vi "Playback Controls.vi"() -> ()   [LabVIEW 2014]
uses:
  <vilib>/Rock Robotics/WPI/Dashboard/WPI_DashboardPlay Operation.ctl
  <vilib>/Rock Robotics/WPI/Dashboard/WPI_DashboardLogging Global.vi
  <vilib>/Utility/inputDevices.llb/mouseAcquire.vi
panel:
  in  "Operation":u16(ring) items=["", "Rename", "Delete", "Show Folder"]
  in  "Rename":string
  in  "Dragging?":bool
  in  "Scrollbar":dbl(slide) scale=0.0..3.043
  in  "Speed":u16(ring)=3 items=["1/10 x", "1/5 x", "1/2 x", "1 x", "2 x", "5 x", "10 x"]
  in  "Playback Button":bool
  in  "Pause Button":bool
  in  "File Selector":u16(ring) items=["Select a Log File", "2013_08_04 10_32_21 Sun -- 1.2 secs", "2013_08_04 10_32_23 Sun -- 0.6 secs", "2013_08_04 10_32_25 Sun -- 0.6 secs", "2013_08_04 10_32_26 Sun -- 0.5 secs", "2013_08_04 10_32_28 Sun -- 0.7 secs", "2013_08_04 10_32_29 Sun -- 0.7 secs", "2013_08_04 10_32_31 Sun -- 0.5 secs", "2013_08_04 10_32_32 Sun -- 14.4 secs", "bar -- 2.2 secs", "foo -- 3.0 secs"]
  in  "Drag Button":bool
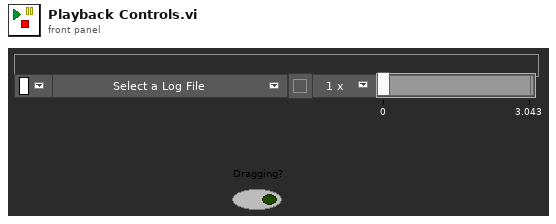
[diagram p1: front panel]
types:
  T1 = typedef "WPI_DashboardPlay Operation.ctl" = enum16{"Play", "Pause", "Finished"}
  T2 = typedef "LVRectTypeDef.ctl" = cluster{"Left":i16, "Top":i16, "Right":i16, "Bottom":i16}
  T3 = cluster{"Horizontal":i32, "Vertical":i32, "Scrolling":i32}
  T4 = cluster{"Horizontal":i32, "Vertical":i32, "Horizontal":i32, "Vertical":i32}
  T5 = cluster{"button 1":bool, "button 2":bool, "button 3":bool, "button 4":bool}
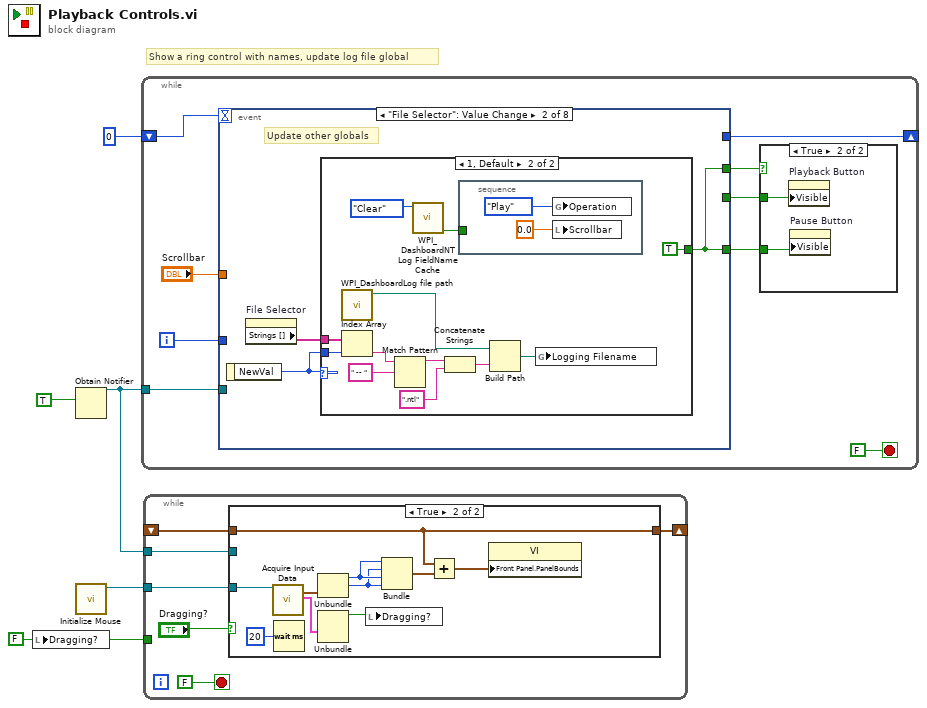
[diagram p0: block diagram]
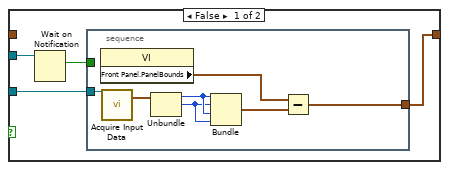
[diagram p2: hidden frame]
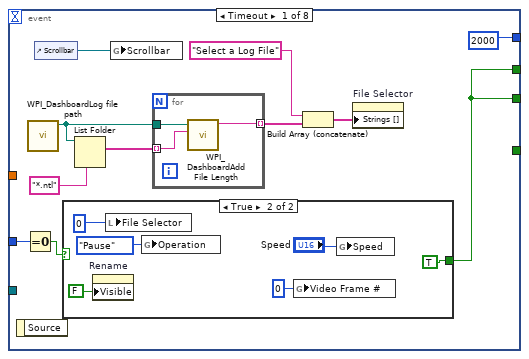
[diagram p4: hidden frame]
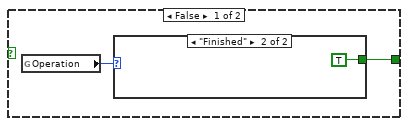
[diagram p5: hidden frame]
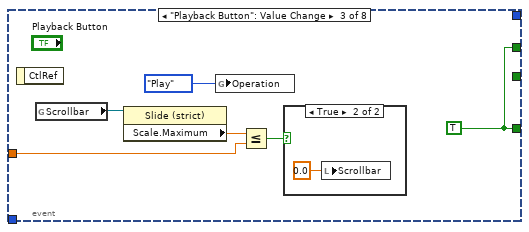
[diagram p8: hidden frame]
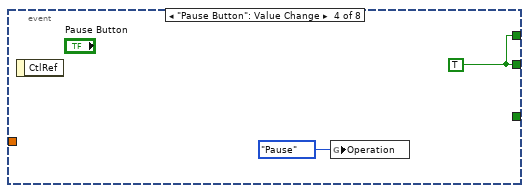
[diagram p10: hidden frame]
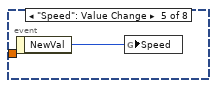
[diagram p11: hidden frame]
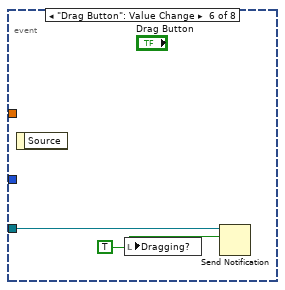
[diagram p12: hidden frame]
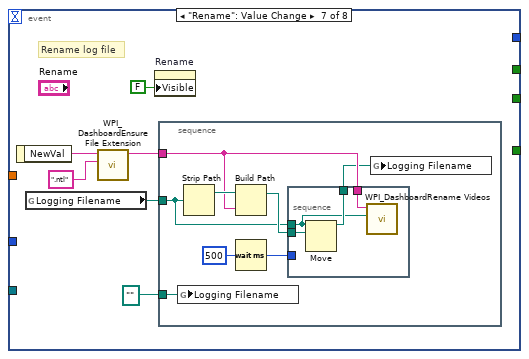
[diagram p13: hidden frame]
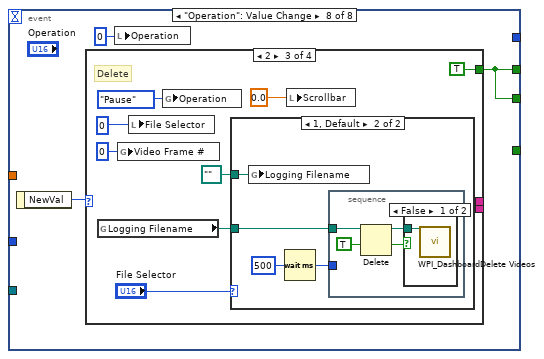
[diagram p14: hidden frame]
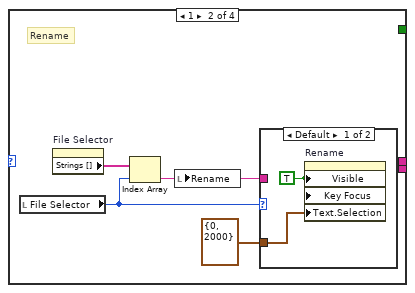
[diagram p16: hidden frame]
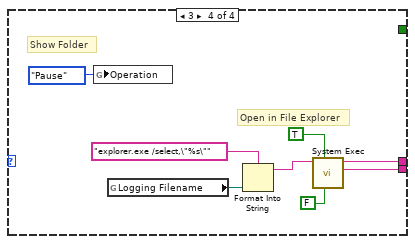
[diagram p20: hidden frame]
diagram:
  w2 = FALSE ("Dragging?")
  # "Show a ring control with names, update log file global"
  n1 = local write "Dragging?"(w2) -> ()
  n2 = Obtain Notifier(notification data type=TRUE ("Dragging?")) -> (notifier out=w3:refnum<notifier>)  [unwired: 3 in, 2 out]
  n3 = call <vilib>:"Initialize Mouse.vi"() -> ("device ID"=w4:refnum<k1>)  [unwired: 10 in, 1 out]
  n4 = while {
    shift-right: [w13] -> _
    shift-left: 0 -> [w12]
    tunnel: w3 -> [w6]
    i -> [w8]
    stop <- FALSE stop-if-true
    n5 = event shown="[1] \"File Selector\": Value Change" {
      selector: _ -> [_ _ _ _ _ _ _ _]
      dyn-events: _ -> [_ _ _ _ _ _ _ _]
      timeout: w12 -> [_ _ _ _ _ _ _ _]
      tunnel: [2000 _ _ _ _ _ _ _] -> w13
      tunnel: [_ w40 w62 _ _ _ _ _] -> w11
      tunnel: [w18 _ _ w65 _ _ _ w88] -> w10
      tunnel: [w18 w40 w62 w65 _ _ _ w88] -> w9
      tunnel: w8 -> [w20 _ _ _ _ _ _ _]
      tunnel: "Scrollbar" -> [_ _ w58 _ _ _ _ _]
      tunnel: w6 -> [_ _ _ _ _ w68 _ _]
      event Timeout {
        n6 = event-data() -> ()  [unwired: 1 in, 1 out]
        n7 = Equal To 0?(x=w20) -> (x = 0?=w19:bool)
        n8 = call <vilib>:"WPI_DashboardLog file path.vi"() -> ("appended path"=w17:path)  [unwired: 11 in]
        n9 = control-ref of="Scrollbar"() -> (w24:refnum<vi>)
        n10 = case shown="True" w19 {
          tunnel: [w28 TRUE] -> w18
          frame False {
            n11 = global read "WPI_DashboardLogging Global.vi" "Operation"() -> (w29:T1)
            n12 = case shown="\"Finished\"" w29 {
              tunnel: [_ TRUE] -> w28
              frame Default {
              }
              frame "Finished" {
              }
            }
          }
          frame True {
            n13 = property on="Rename" class="Str"("Visible"=FALSE) -> ()  [unwired: 2 in, 2 out]
            n14 = local write "File Selector"(0) -> ()
            n15 = global write "WPI_DashboardLogging Global.vi" "Operation"(WPI_DashboardPlay_Operation."Pause" ("Operation")) -> ()
            n16 = global write "WPI_DashboardLogging Global.vi" "Video Frame #"(0 ("Video Frame #")) -> ()
            n17 = global write "WPI_DashboardLogging Global.vi" "Speed"("Speed") -> ()
          }
        }
        n18 = List Folder(path=w17, pattern="*.ntl") -> (filenames=w26:string[])  [unwired: 2 in, 3 out]
        n19 = global write "WPI_DashboardLogging Global.vi" "Scrollbar"(w24) -> ()
        n20 = for {
          tunnel: w26 -> [w37] mode=indexing
          tunnel: [w39] -> w23 mode=indexing
          tunnel: w17 -> [w38]
          n21 = call <vilib>:"WPI_DashboardAdd File Length.vi"("String in"=w37, "appended path"=w38) -> ("String out"=w39:string)  [unwired: 9 in]
        }
        n22 = Build Array (concatenate)("Select a Log File" ("pattern"), w23) -> (w22:string[])
        n23 = property on="File Selector" class="Ring (strict)"("Strings []"=w22) -> ()  [unwired: 2 in, 2 out]
      }
      event "File Selector": Value Change {
        # "Update other globals"
        n24 = event-data() -> ("NewVal"=w41:u16)  [unwired: 1 in]
        n25 = property on="File Selector" class="Ring (strict)"() -> ("Strings []"=w42:string[])  [unwired: 2 in, 2 out]
        n26 = case shown="1, Default" w41 {
          tunnel: w42 -> [_ w54]
          tunnel: w41 -> [_ w53]
          tunnel: [_ TRUE ("Visible")] -> w40
          frame 0 {
          }
          frame 1, Default {
            n27 = call <vilib>:"WPI_DashboardLog file path.vi"() -> ("appended path"=w52:path)  [unwired: 11 in]
            n28 = Index Array(array=w54, index=w53) -> (element=w48:string)
            n29 = Match Pattern(string=w48, regular expression=" -- ") -> (before substring=w43:string)  [unwired: 1 in, 3 out]
            n30 = call <vilib>:"WPI_DashboardNT Log FieldName Cache.vi"("Operation"=enum16{"Lookup/Add", "Index", "Clear"}."Clear") -> ("New/Valid"=w45:bool)  [unwired: 8 in, 2 out]
            n31 = Concatenate Strings(w43, ".ntl") -> (w50:string)
            n32 = stacked-sequence {
              tunnel: w45 -> [_]
              frame #0 {
                n33 = global write "WPI_DashboardLogging Global.vi" "Operation"(WPI_DashboardPlay_Operation."Play" ("Operation")) -> ()
                n34 = local write "Scrollbar"(0.0 ("Position")) -> ()
              }
            }
            n35 = Build Path(base path=w52, name or relative path=w50) -> (appended path=w49:path)
            n36 = global write "WPI_DashboardLogging Global.vi" "Logging Filename"(w49) -> ()
          }
        }
      }
      event "Playback Button": Value Change {
        w62 = TRUE ("Visible")
        n37 = event-data() -> ()  [unwired: 1 in, 1 out]
        n38 = global read "WPI_DashboardLogging Global.vi" "Scrollbar"() -> (w60:refnum<vi>)
        n39 = property class="Slide (strict)"(reference=w60) -> ("Scale.Maximum"=w59:dbl)  [unwired: 1 in, 2 out]
        n40 = global write "WPI_DashboardLogging Global.vi" "Operation"(WPI_DashboardPlay_Operation."Play" ("Operation")) -> ()
        n41 = Less Or Equal?(x=w59, y=w58) -> (x <= y?=w57:bool)
        n42 = case shown="True" w57 {
          frame False {
          }
          frame True {
            n43 = local write "Scrollbar"(0.0 ("Scrollbar")) -> ()
          }
        }
      }
      event "Pause Button": Value Change {
        w65 = TRUE ("Visible")
        n44 = event-data() -> ()  [unwired: 1 in, 1 out]
        n45 = global write "WPI_DashboardLogging Global.vi" "Operation"(WPI_DashboardPlay_Operation."Pause" ("Operation")) -> ()
      }
      event "Speed": Value Change {
        n46 = event-data() -> ("NewVal"=w66:u16)  [unwired: 1 in]
        n47 = global write "WPI_DashboardLogging Global.vi" "Speed"(w66) -> ()
      }
      event "Drag Button": Value Change {
        w67 = TRUE ("Dragging?")
        n48 = event-data() -> ()  [unwired: 1 in, 1 out]
        n49 = local write "Dragging?"(w67) -> ()
        n50 = Send Notification(notification=w67, notifier=w68) -> ()  [unwired: 1 in, 2 out]
      }
      event "Rename": Value Change {
        # "Rename log file"
        n51 = event-data() -> ("NewVal"=w71:string)  [unwired: 1 in]
        n52 = global read "WPI_DashboardLogging Global.vi" "Logging Filename"() -> (w73:path)
        n53 = call <vilib>:"WPI_DashboardEnsure File Extension.vi"("Extension"=".ntl", "Name"=w71) -> ("Name Out"=w70:string)  [unwired: 9 in]
        n54 = property on="Rename" class="Str"("Visible"=FALSE) -> ()  [unwired: 2 in, 2 out]
        n55 = stacked-sequence {
          tunnel: w70 -> [w76]
          tunnel: w73 -> [w80]
          tunnel: path "" ("Logging Filename") -> [w79]
          frame #0 {
            n56 = global write "WPI_DashboardLogging Global.vi" "Logging Filename"(w79) -> ()
            n57 = Strip Path(path=w80) -> (stripped path=w82:path)  [unwired: 1 out]
            n58 = Build Path(base path=w82, name or relative path=w76) -> (appended path=w81:path)
            n59 = Wait (ms)(milliseconds to wait=u32 500) -> (millisecond timer value=w77:u32)
            n60 = stacked-sequence {
              tunnel: w81 -> [w86]
              tunnel: w80 -> [w83]
              tunnel: w77 -> [_]
              tunnel: w76 -> [w85]
              tunnel: [w84] -> w75
              frame #0 {
                n61 = Move(source path=w83, 10:w86) -> (3:w84:path)  [unwired: 3 in, 2 out]
                n62 = call <vilib>:"WPI_DashboardRename Videos.vi"("Path"=w83, "Log Name"=w85) -> ()  [unwired: 10 in]
              }
            }
            n63 = global write "WPI_DashboardLogging Global.vi" "Logging Filename"(w75) -> ()
          }
        }
      }
      event "Operation": Value Change {
        n64 = event-data() -> ("NewVal"=w89:u16)  [unwired: 1 in]
        n65 = case shown="2" w89 {
          tunnel: [_ _ TRUE _] -> w88
          tunnel: [_ _ _ w116] -> _
          tunnel: [_ _ _ w115] -> _
          frame 0, Default {
          }
          frame 1 {
            # "Rename"
            n66 = local read "File Selector"() -> (w91:u16)
            n67 = property on="File Selector" class="Ring (strict)"() -> ("Strings []"=w93:string[])  [unwired: 2 in, 2 out]
            n68 = Index Array(array=w93, index=w91) -> (element=w92:string)
            n69 = local write "Rename"(w92) -> ()
            n70 = case shown="Default" w91 {
              tunnel: w92 -> [_ _]
              tunnel: cluster{i32, i32} {0, 2000} -> [w94 _]
              frame Default {
                w95 = TRUE ("Visible")
                n71 = property on="Rename" class="Str"("Visible"=w95, "Key Focus"=w95, "Text.Selection"=w94) -> ()  [unwired: 2 in, 2 out]
              }
              frame 0 {
              }
            }
          }
          frame 2 {
            # "Delete"
            n72 = global read "WPI_DashboardLogging Global.vi" "Logging Filename"() -> (w98:path)
            n73 = global write "WPI_DashboardLogging Global.vi" "Video Frame #"(0 ("Video Frame #")) -> ()
            n74 = local write "File Selector"(0) -> ()
            n75 = global write "WPI_DashboardLogging Global.vi" "Operation"(WPI_DashboardPlay_Operation."Pause" ("Operation")) -> ()
            n76 = case shown="1, Default" "File Selector" {
              tunnel: w98 -> [_ w107]
              tunnel: path "" ("Logging Filename") -> [_ w106]
              frame 0 {
              }
              frame 1, Default {
                n77 = global write "WPI_DashboardLogging Global.vi" "Logging Filename"(w106) -> ()
                n78 = Wait (ms)(milliseconds to wait=u32 500) -> (millisecond timer value=w104:u32)
                n79 = stacked-sequence {
                  tunnel: w107 -> [w111]
                  tunnel: w104 -> [_]
                  frame #0 {
                    n80 = Delete(path (use dialog)=w111, confirm (F)=TRUE) -> (deleted path=w108:path, cancelled=w109:bool)  [unwired: 3 in, 1 out]
                    n81 = case shown="False" w109 {
                      tunnel: w108 -> [w112 _]
                      frame False {
                        n82 = call <vilib>:"WPI_DashboardDelete Videos.vi"("Path"=w112) -> ()  [unwired: 11 in]
                      }
                      frame True {
                      }
                    }
                  }
                }
              }
            }
            n83 = local write "Scrollbar"(0.0 ("Position")) -> ()
          }
          frame 3 {
            # "Open in File Explorer"
            # "Show Folder"
            n84 = global write "WPI_DashboardLogging Global.vi" "Operation"(WPI_DashboardPlay_Operation."Pause" ("Operation")) -> ()
            n85 = global read "WPI_DashboardLogging Global.vi" "Logging Filename"() -> (w113:path)
            n86 = Format Into String(format string="explorer.exe /select,\"%s\"", w113) -> (resulting string=w119:string)  [unwired: 2 in, 1 out]
            n87 = call <vilib>:"System Exec.vi"("run minimized? (F)"=FALSE, "wait until completion? (T)"=TRUE, "command line"=w119) -> ("standard error"=w116:string, "standard output"=w115:string)  [unwired: 5 in, 2 out]
          }
        }
        n88 = local write "Operation"(0) -> ()
      }
    }
    n89 = case shown="True" w9 {
      tunnel: w11 -> [_ w16]
      tunnel: w10 -> [_ w15]
      frame False {
      }
      frame True {
        n90 = property on="Playback Button" class="Bool"("Visible"=w15) -> ()  [unwired: 2 in, 2 out]
        n91 = property on="Pause Button" class="Bool"("Visible"=w16) -> ()  [unwired: 2 in, 2 out]
      }
    }
  }
  n92 = while {
    tunnel: w4 -> [w126]
    tunnel: w3 -> [w124]
    tunnel: w2 -> [_]
    shift-right: [w122] -> _
    shift-left: _ -> [w121]
    stop <- FALSE stop-if-true
    n93 = case shown="True" "Dragging?" {
      tunnel: w126 -> [w129 w147]
      tunnel: w124 -> [w130 _]
      tunnel: [w128 w139] -> w122
      tunnel: w121 -> [_ w139]
      frame False {
        n94 = Wait on Notification(notifier=w130) -> (notification=w127:bool)  [unwired: 3 in, 3 out]
        n95 = stacked-sequence {
          tunnel: w129 -> [w137]
          tunnel: [w133] -> w128
          tunnel: w127 -> [_]
          frame #0 {
            n96 = property class="VI"() -> ("Front Panel.PanelBounds"=w135:T2)  [unwired: 2 in, 2 out]
            n97 = call-poly <vilib>:"Acquire Input Data.vi"("device ID"=w137) -> ("axis info"=w136:T3)  [unwired: 15 in, 3 out]
            n98 = Unbundle(w136) -> ("Horizontal"=w132:i32, "Vertical"=w131:i32)  [unwired: 1 out]
            n99 = Bundle("Horizontal"=w132, "Vertical"=w131, "Horizontal"=w132, "Vertical"=w131) -> (w134:T4)  [unwired: 1 in]
            n100 = Subtract(x=w135, y=w134) -> (x-y=w133:cluster{i32, i32, i32, i32})
          }
        }
      }
      frame True {
        n101 = call-poly <vilib>:"Acquire Input Data.vi"("device ID"=w147) -> ("axis info"=w143:T3, "button info"=w145:T5)  [unwired: 15 in, 2 out]
        n102 = Wait (ms)(milliseconds to wait=u32 20) -> ()  [unwired: 1 out]
        n103 = Unbundle(w143) -> ("Horizontal"=w142:i32, "Vertical"=w141:i32)  [unwired: 1 out]
        n104 = Unbundle(w145) -> ("button 1"=w144:bool)  [unwired: 3 out]
        n105 = local write "Dragging?"(w144) -> ()
        n106 = Bundle("Horizontal"=w142, "Vertical"=w141, "Horizontal"=w142, "Vertical"=w141) -> (w140:T4)  [unwired: 1 in]
        n107 = Add(x=w139, y=w140) -> (x+y=w138:cluster{i32, i32, i32, i32})
        n108 = property class="VI"("Front Panel.PanelBounds"=w138) -> ()  [unwired: 2 in, 2 out]
      }
    }
  }
